vi "image2data_2d.vi"(10 "image_1d":sgl[](array[numeric]), 11 "Data":T1 {"slice orientation" items=["transverse unflipped", "coronal unflipped", "sagittal unflipped", "transverse flipped", "coronal flipped", "sagittal flipped"]}) -> (2 "imag2_2d":sgl[][](array[numeric]), 3 "Data":T1 {"slice orientation" items=["transverse unflipped", "coronal unflipped", "sagittal unflipped", "transverse flipped", "coronal flipped", "sagittal flipped"]})   [LabVIEW 2014]
uses:
  control/head_data.ctl
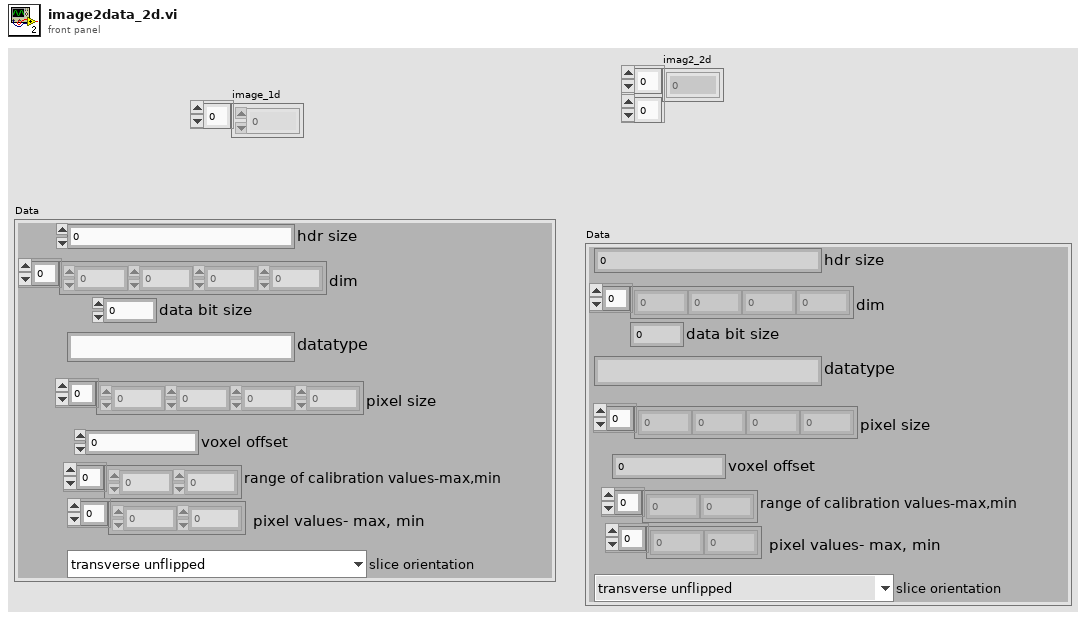
[diagram p1: front panel]
types:
  T1 = typedef "head_data.ctl" = cluster{"hdr size":i32, "dim":i32[], "data bit size":i32, "datatype":string, "pixel size ":sgl[], "voxel offset":sgl, "range of calibration values-max,min":sgl[], " pixel values- max, min":sgl[], "slice orientation":u16}
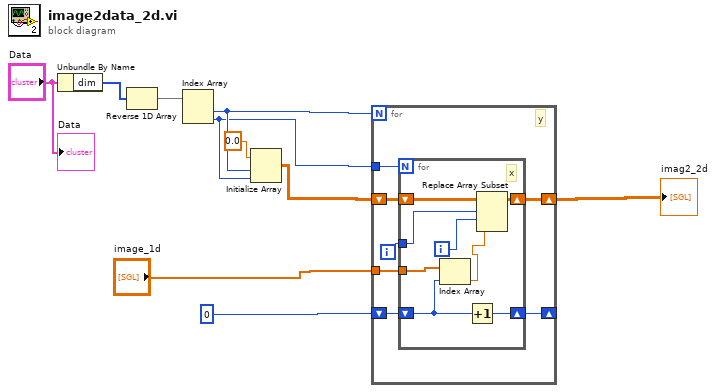
[diagram p0: block diagram]
diagram:
  n1 = Unbundle By Name("Data") -> ("dim"=w2:i32[])
  n2 = Reverse 1D Array(array=w2) -> (reversed array=w1:i32[])
  n3 = Index Array(array=w1) -> (element #1=w7:i32, element #2=w6:i32)  [unwired: 2 in]
  n4 = Initialize Array(sgl 0.0 ("element"), w7, w6) -> (w4:sgl[][])
  n5 = for {
    N: w7 -> [_]
    tunnel: "image_1d" -> [w17]
    shift-right: [w16] -> _
    shift-left: 0 -> [w15]
    tunnel: w6 -> [w14]
    shift-right: [w12] -> w3
    shift-left: w4 -> [w13]
    i -> [w11]
    # "y"
    n6 = for {
      N: w14 -> [_]
      tunnel: w17 -> [w25]
      shift-right: [w24] -> w16
      shift-left: w15 -> [w23]
      shift-right: [w21] -> w12
      shift-left: w13 -> [w22]
      tunnel: w11 -> [w19]
      i -> [w18]
      # "x"
      n7 = Index Array(array=w25, index=w23) -> (element=w20:sgl)
      n8 = Increment(x=w23) -> (x+1=w24:i32)
      n9 = Replace Array Subset(array=w22, new element=w20, index (row)=w19, index (col)=w18) -> (w21:sgl[][])
    }
  }
  "imag2_2d" <- w3
  "Data" <- "Data"
